vi "Read Description.vi"(11 "Mocha in":refnum<class "Mocha.lvclass">) -> (2 "Description":string, 3 "Mocha out":refnum<class "Mocha.lvclass">)   [LabVIEW 2020, in "Mocha.lvclass"]
uses:
  Mocha.lvclass
  Mocha.lvclass/Mocha.ctl
  Beverage.lvclass
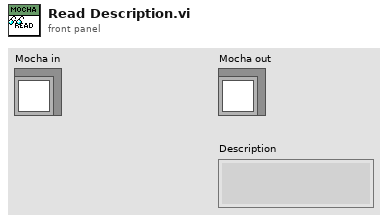
[diagram p1: front panel]
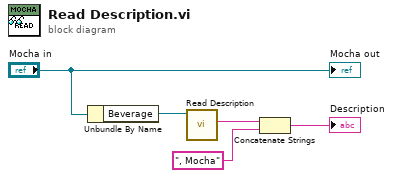
[diagram p0: block diagram]
diagram:
  n1 = Unbundle By Name("Mocha in") -> ("Beverage"=w4:refnum<class "Beverage.lvclass">)
  n2 = call-dynamic "Read Description.vi"("Beverage in"=w4) -> ("Description"=w3:string)  [unwired: 9 in, 1 out]
  n3 = Concatenate Strings(w3, ", Mocha" ("string")) -> (→"Description":string)
  "Mocha out" <- "Mocha in"
